vi "Instantiate.vi"(0 "py session":refnum<k35>, 5 "Ticker":string, 11 "error in":errorcluster) -> (4 "lvFinanceFunctionsHL out":refnum<class "lvFinanceFunctionsHL.lvclass">, 15 "error out":errorcluster)   [LabVIEW 2020, in "lvFinanceFunctionsHL.lvclass"]
uses:
  lvFinanceFunctionsHL.lvclass
  lvFinanceFunctionsHL.lvclass/lvFinanceFunctionsHL.ctl
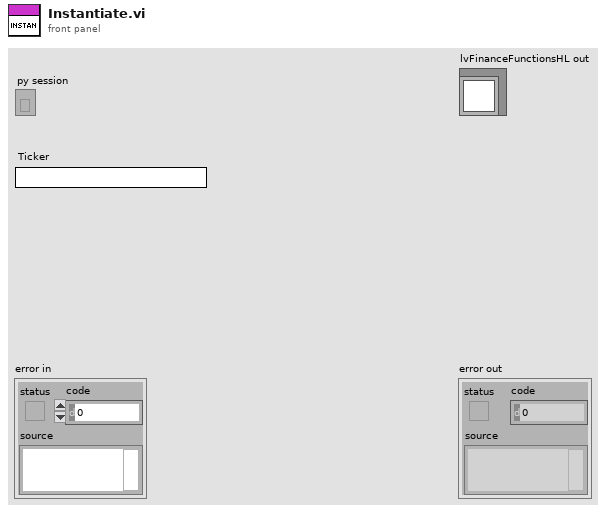
[diagram p1: front panel]
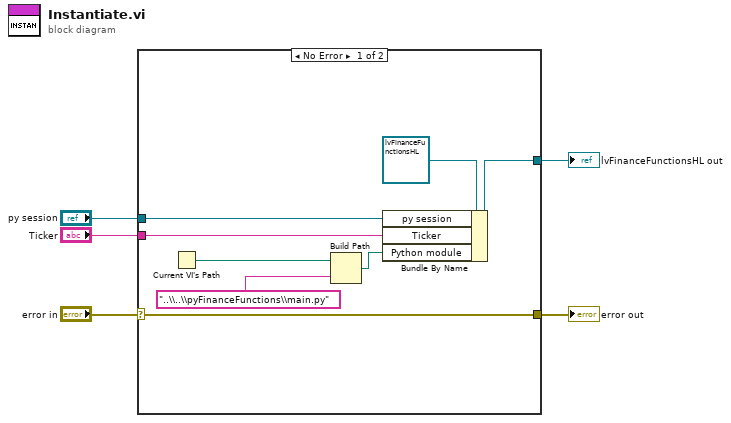
[diagram p0: block diagram]
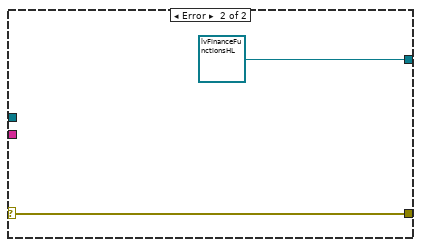
[diagram p2: hidden frame]
diagram:
  n1 = case shown="No Error" "error in" {
    selector: "error in" -> [w13 w15]
    tunnel: [w13 w15] -> w4
    tunnel: "Ticker" -> [w11 _]
    tunnel: [w10 refnum<class "lvFinanceFunctionsHL.lvclass"> refnum ("lvFinanceFunctionsHL out")] -> w2
    tunnel: "py session" -> [w9 _]
    frame No Error {
      n2 = Current VI's Path() -> (path=w8:path)
      n3 = Build Path(base path=w8, name or relative path="..\\..\\pyFinanceFunctions\\main.py") -> (appended path=w6:path)
      n4 = Bundle By Name(cluster=refnum<class "lvFinanceFunctionsHL.lvclass"> refnum ("lvFinanceFunctionsHL out"), "py session"=w9, "Ticker"=w11, "Python module"=w6) -> (w10:refnum<class "lvFinanceFunctionsHL.lvclass">)
    }
    frame Error {
    }
  }
  "error out" <- w4
  "lvFinanceFunctionsHL out" <- w2
